vi "MwE with Feeder-.vi"() -> ()   [LabVIEW 2016]
doc: "This example shows how to move a motor connected to an encoder and a wheel, and then read information about the system from an encoder.\n\nThis is an example of how to use feedback (from the encoder) to create an open loop system. If some control method was used, for example using PID, a closed loop system could be created.\n\nThis example expects a USB cable connected from your development PC to the Type B USB Jack (next to the power input) on the roboRIO.\n\nThis example requires the Driver Station to be running with Teleoperated Enabled."
uses:
  <vilib>/Rock Robotics/SystemInterfaces/DIO/FPGA_DIOChannel.ctl
  <vilib>/Rock Robotics/WPI/Encoder/WPI_EncoderType.ctl
  <vilib>/Rock Robotics/SystemInterfaces/DIO/FPGA_DIOPWMChannel.ctl
  <vilib>/Rock Robotics/WPI/MotorControl/WPI_MotorControlOpen SPARK.vi
  <vilib>/Rock Robotics/WPI/Counter/WPI_CounterDigitalInputToDigitalSource.vi
  <vilib>/gmath/NI_Gmath.lvlib
panel:
  in  "Feeder Enabled":bool=TRUE
  out "RPM F":cluster{dbl, dbl}[](graph)
  in  "Motor PWM Channel F":T1=enum."PWM 8"
  in  "Number Samples to Average F":u8=1 min=1 max=128
  in  "Invert Direction F":bool=TRUE
  in  "Decoding Type F":T2=enum."2x"
  in  "DistancePerCount (deg) F":dbl=0.351563
  in  "Encoder B Channel F":T3=enum."DIO 3"
  in  "Encoder A Channel F":T3=enum."DIO 2"
  in  "Minimum Rate F":dbl=20.0
  in  "Update RPM F":bool
  in  "Target RPM F":dbl=770.0
  out "DS Original F":dbl=0.6428571428571428
  in  "Lower Limit F":dbl=-50.0 format="%#_13g"
  in  "Upper Limit F":dbl=50.0 format="%#_13g"
  in  "Pos Drive Signal F":dbl=0.4
  in  "Neg Drive Signal F":dbl=0.05
  out "Error F":dbl(graph)=-19.827905182603445
  out "Error F":dbl=-19.827905182603445
  out "RPM F":dbl=3319.8279051826034
  out "RPM F":dbl(graph)=3319.8279051826034
  out "Encoder Alarm Status F":string="Encoder Moving"
  out "Encoder Direction F":string="Forward"
  in  "Encoder Before Gearbox":bool
  in  "Update RPM L":bool
  in  "Lower Limit L":dbl=-50.0 format="%#_13g"
  in  "Upper Limit L":dbl=50.0 format="%#_13g"
  out "Error L":dbl(graph)=-19.827905182603445
  out "Error L":dbl=-19.827905182603445
  out "DS Original L":dbl=0.6428571428571428
  in  "Neg Drive Signal":dbl=0.6
  in  "Pos Drive Signal":dbl=1.0
  in  "Target RPM":dbl=3300.0
  in  "MS to Wait":u32=10
  out "Loop Time (s)":dbl=0.010378 format="%_6f"
  out "RPM L":dbl=3319.8279051826034
  out "RPM":cluster{dbl[], dbl[]}[](graph)
  out "RPM L":dbl(graph)=3319.8279051826034
  in  "Motor PWM Channel":T1=enum."PWM 9"
  in  "Number Samples to Average":u8=1 min=1 max=128
  in  "Invert Direction L":bool=TRUE
  in  "Decoding Type":T2=enum."2x"
  in  "DistancePerCount (deg)":dbl=0.351563
  in  "Encoder B Channel":T3=enum."DIO 1"
  in  "Encoder A Channel":T3
  in  "Minimum Rate":dbl=20.0
  in  "Stop":bool
  out "Encoder Alarm Status L":string="Encoder Moving"
  out "Encoder Direction L":string="Forward"
  # "These can be set while running."
  # "Output information."
  # "Set these inputs before running."
  # "This example requires the Driver Station to be running with Teleoperated Enabled."
  # "Need to tune target RPM and drive signals"
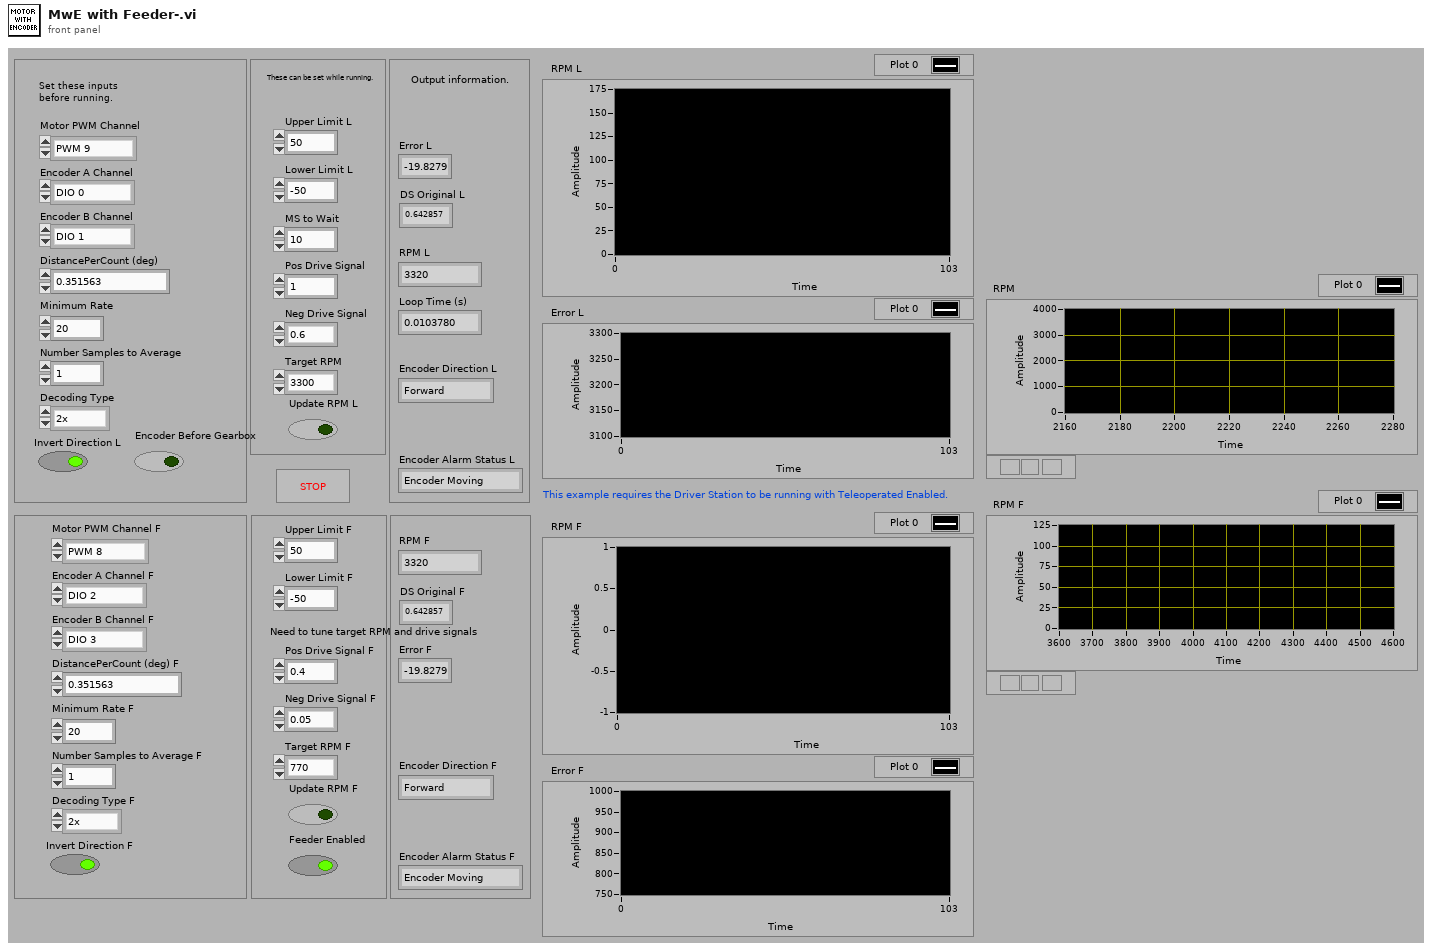
[diagram p1: front panel]
types:
  T1 = typedef "FPGA_DIOPWMChannel.ctl" = enum8{"PWM 0", "PWM 1", "PWM 2", "PWM 3", "PWM 4", "PWM 5", "PWM 6", "PWM 7", "PWM 8", "PWM 9", "PWM MXP 0", "PWM MXP 1", "PWM MXP 2", "PWM MXP 3", "PWM MXP 4", "PWM MXP 5", "PWM MXP 6", "PWM MXP 7", "PWM MXP 8", "PWM MXP 9", "Invalid"}
  T2 = typedef "WPI_EncoderType.ctl" = enum16{"1x", "2x", "4x"}
  T3 = typedef "FPGA_DIOChannel.ctl" = enum8{"DIO 0", "DIO 1", "DIO 2", "DIO 3", "DIO 4", "DIO 5", "DIO 6", "DIO 7", "DIO 8", "DIO 9", "DIO MXP 0", "DIO MXP 1", "DIO MXP 2", "DIO MXP 3", "DIO MXP 4", "DIO MXP 5", "DIO MXP 6", "DIO MXP 7", "DIO MXP 8", "DIO MXP 9", "DIO MXP 10", "DIO MXP 11", "DIO MXP 12", "DIO MXP 13", "DIO MXP 14", "DIO MXP 15", "SPI Port CS1", "SPI Port CS2", "SPI Port CS3", "SPI Port MISO", "SPI Port MOSI", "Invalid"}
  T4 = typedef "WPI_DigitalInputDevRef.ctl" = cluster{"DevStatus":errorcluster, "DIO Channel":T3}
  T5 = typedef "WPI_MotorControlDeviceRef.ctl" = cluster{"DeviceStatus":errorcluster, "Type":T6, "PWM":cluster{"PWM Channel":T1, "DeadBand":T7}, "CAN":cluster{"Device Number":u8, "SetOutput VI Ref":variant, "GetOutput VI Ref":variant, "Enable VI Ref":variant, "Disable VI Ref":variant, "Data":variant}, "Invert":bool}
  T6 = typedef "WPI_MotorControlType.ctl" = enum16{"PWM", "CAN"}
  T7 = typedef "WPI_PWMDeadband.ctl" = cluster{"Name":string, "maxPositivePwm":i32, "minPositivePwm":i32, "centerPwm":i32, "maxNegativePwm":i32, "minNegativePwm":i32, "angularRange":u16}
  T8 = typedef "FPGA_CounterEncoderSourceConvertionLVSourceType.ctl" = cluster{"DevStatus":errorcluster, "AnalogTriggerMode?":bool, "DigitalMode":cluster{"DIO Channel":T9}, "AnalogTriggerMode":cluster{"AnalogTriggerIndex":T10, "OutputType":T11}}
  T9 = typedef "FPGA_DIODigitalSourceChannel.ctl" = enum8{"DIO 0", "DIO 1", "DIO 2", "DIO 3", "DIO 4", "DIO 5", "DIO 6", "DIO 7", "DIO 8", "DIO 9", "DIO MXP 0", "DIO MXP 1", "DIO MXP 2", "DIO MXP 3", "DIO MXP 4", "DIO MXP 5", "DIO MXP 6", "DIO MXP 7", "DIO MXP 8", "DIO MXP 9", "DIO MXP 10", "DIO MXP 11", "DIO MXP 12", "DIO MXP 13", "DIO MXP 14", "DIO MXP 15", "Disabled"}
  T10 = typedef "FPGA_AnalogTriggerIndex.ctl" = enum8{"Trig 0", "Trig 1", "Trig 2", "Trig 3", "Trig 4", "Trig 5", "Trig 6", "Trig 7", "Invalid"}
  T11 = typedef "FPGA_AnalogTriggerOutType.ctl" = enum16{"InWindow", "TriggerState", "Rising", "Falling"}
  T12 = typedef "WPI_EncoderDevRef.ctl" = cluster{"DevStatus":errorcluster, "EncoderIndex":T13, "CounterIndex":T14, "DistancePerCount":dbl, "Decoding Type":T2}
  T13 = typedef "FPGA_EncoderIdx.ctl" = enum8{"Enc 0", "Enc 1", "Enc 2", "Enc 3", "Enc 4", "Enc 5", "Enc 6", "Enc 7", "Invalid"}
  T14 = typedef "FPGA_CounterCtrSystemIndex.ctl" = enum8{"Ctr 0", "Ctr 1", "Ctr 2", "Ctr 3", "Ctr 4", "Ctr 5", "Ctr 6", "Ctr 7", "Invalid"}
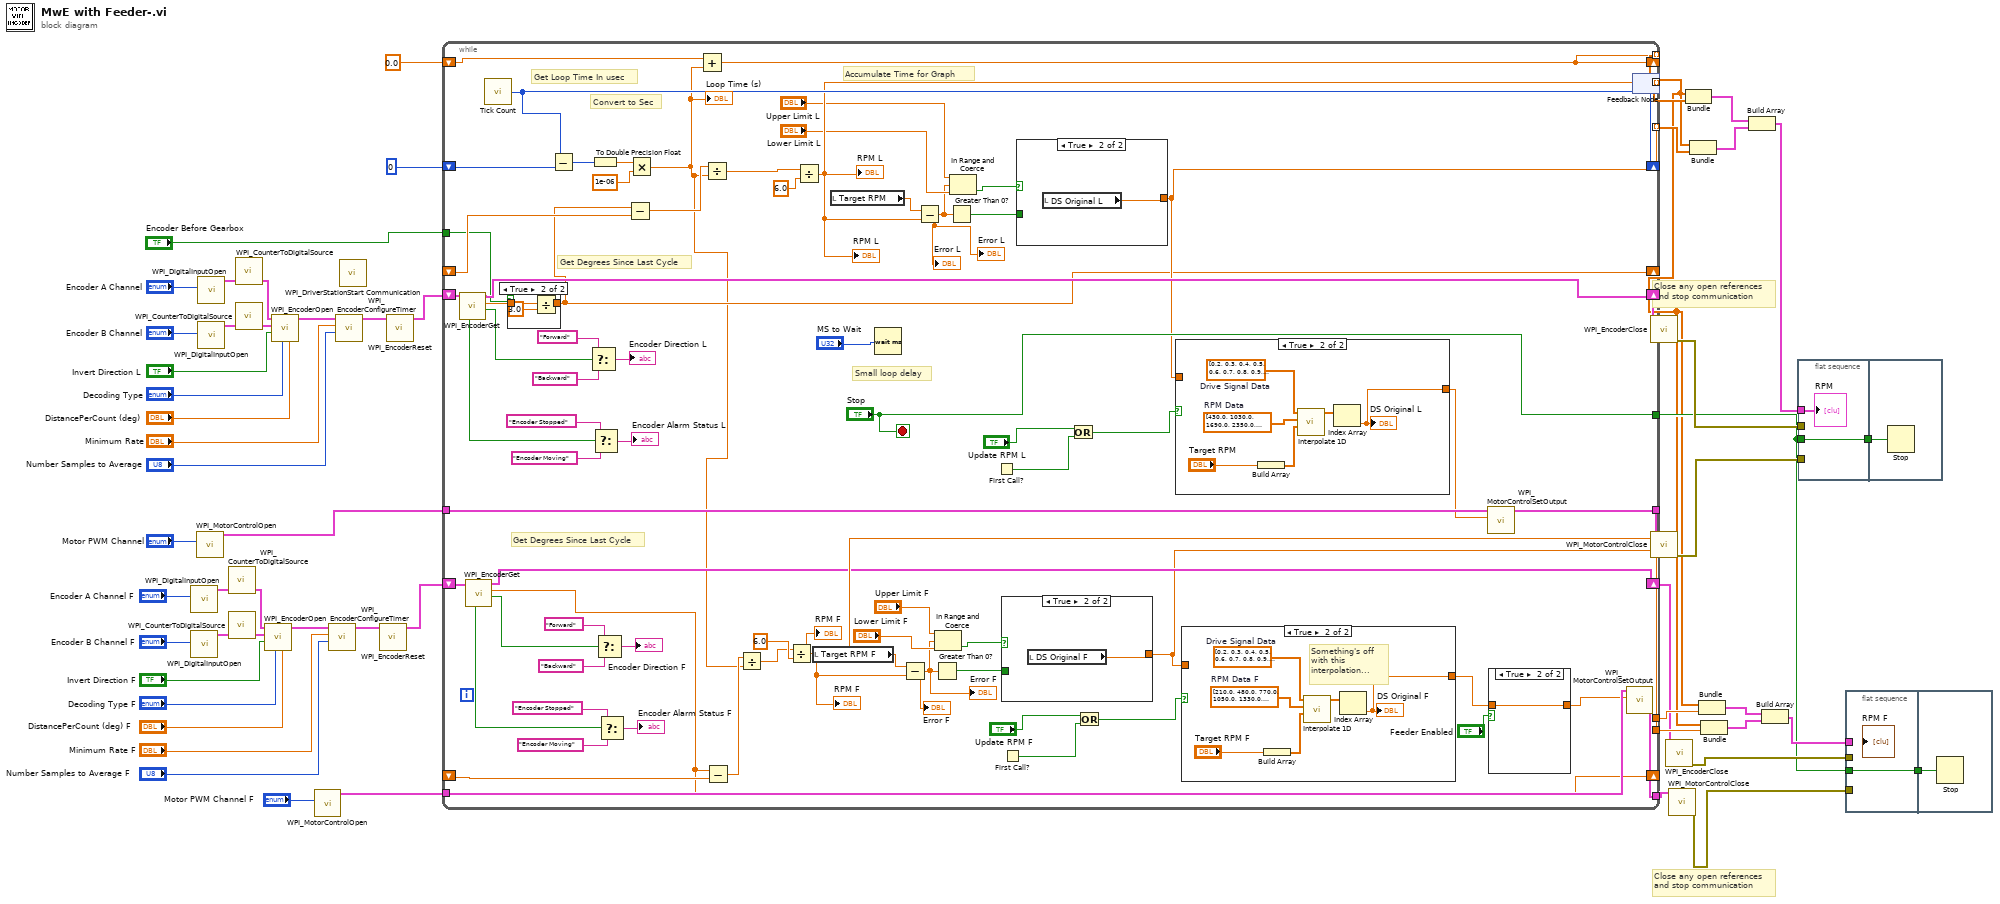
[diagram p0: block diagram]
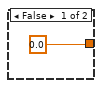
[diagram p2: hidden frame]
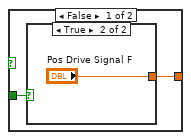
[diagram p4: hidden frame]
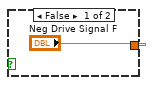
[diagram p5: hidden frame]
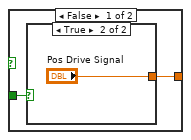
[diagram p8: hidden frame]
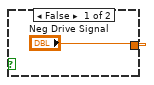
[diagram p9: hidden frame]
diagram:
  # "Close any open references\nand stop communication"
  # "Close any open references\nand stop communication"
  n1 = call <vilib>:"WPI_DigitalInputOpen.vi"("DIO Channel"="Encoder A Channel F") -> ("DigitalInputDevRef"=w27:T4)  [unwired: 1 in, 9 out]
  n2 = call <vilib>:"WPI_DigitalInputOpen.vi"("DIO Channel"="Encoder B Channel F") -> ("DigitalInputDevRef"=w28:T4)  [unwired: 1 in, 9 out]
  n3 = call-poly <vilib>:"WPI_MotorControlOpen.vi"("PWM Channel"="Motor PWM Channel") -> ("MotorControlDeviceRef"=w31:T5)  [unwired: 3 in, 7 out]
  n4 = call <vilib>:"WPI_DigitalInputOpen.vi"("DIO Channel"="Encoder A Channel") -> ("DigitalInputDevRef"=w55:T4)  [unwired: 1 in, 9 out]
  n5 = call <vilib>:"WPI_DigitalInputOpen.vi"("DIO Channel"="Encoder B Channel") -> ("DigitalInputDevRef"=w56:T4)  [unwired: 1 in, 9 out]
  n6 = call-poly <vilib>:"WPI_CounterToDigitalSource.vi"("DigitalInputDevRef"=w27) -> ("Digital Source"=w26:T8)  [unwired: 6 out]
  n7 = call-poly <vilib>:"WPI_CounterToDigitalSource.vi"("DigitalInputDevRef"=w28) -> ("Digital Source"=w29:T8)  [unwired: 6 out]
  n8 = call-poly <vilib>:"WPI_CounterToDigitalSource.vi"("DigitalInputDevRef"=w55) -> ("Digital Source"=w54:T8)  [unwired: 6 out]
  n9 = call-poly <vilib>:"WPI_CounterToDigitalSource.vi"("DigitalInputDevRef"=w56) -> ("Digital Source"=w57:T8)  [unwired: 6 out]
  n10 = call <vilib>:"WPI_EncoderOpen.vi"("DistancePerCount"="DistancePerCount (deg) F", "Decoding Type"="Decoding Type F", "Invert Direction (False)"="Invert Direction F", "BSource"=w29, "ASource"=w26) -> ("EncoderDevRef"=w20:T12)  [unwired: 3 in, 3 out]
  n11 = call <vilib>:"WPI_EncoderOpen.vi"("DistancePerCount"="DistancePerCount (deg)", "Decoding Type"="Decoding Type", "Invert Direction (False)"="Invert Direction L", "BSource"=w57, "ASource"=w54) -> ("EncoderDevRef"=w48:T12)  [unwired: 3 in, 3 out]
  n12 = call-poly <vilib>:"WPI_MotorControlOpen.vi"("PWM Channel"="Motor PWM Channel F") -> ("MotorControlDeviceRef"=w15:T5)  [unwired: 3 in, 7 out]
  n13 = call <vilib>:"WPI_EncoderConfigureTimer.vi"("Number Samples to Average"="Number Samples to Average F", "Minimum Rate"="Minimum Rate F", "EncoderDevRef"=w20) -> ("EncoderDevRef"=w16:T12)  [unwired: 1 in, 7 out]
  n14 = call <vilib>:"WPI_EncoderConfigureTimer.vi"("Number Samples to Average"="Number Samples to Average", "Minimum Rate"="Minimum Rate", "EncoderDevRef"=w48) -> ("EncoderDevRef"=w42:T12)  [unwired: 1 in, 7 out]
  n15 = call <vilib>:"WPI_DriverStationStart Communication.vi"() -> ()  [unwired: 2 in, 10 out]
  n16 = call <vilib>:"WPI_EncoderReset.vi"("EncoderDevRef"=w16) -> ("EncoderDevRef"=w14:T12)  [unwired: 1 in, 9 out]
  n17 = call <vilib>:"WPI_EncoderReset.vi"("EncoderDevRef"=w42) -> ("EncoderDevRef"=w41:T12)  [unwired: 1 in, 9 out]
  n18 = while {
    shift-right: [w116] -> w58
    shift-left: w41 -> [w119]
    tunnel: ["Stop"] -> w4
    tunnel: w31 -> [w122]
    tunnel: [w121] -> w45
    tunnel: [w104] -> w43 mode=indexing
    tunnel: [w106] -> w2 mode=indexing
    shift-right: [w115] -> _
    shift-left: u32 0 ("Tick Count(uSec)") -> [w114]
    shift-right: [w92] -> _
    shift-left: _ -> [w113]
    shift-right: [w106] -> _
    shift-left: 0.0 ("Tick Count(uSec)") -> [w107]
    tunnel: [w98] -> w37 mode=indexing
    tunnel: "Encoder Before Gearbox" -> [w91]
    tunnel: [w70] -> w7
    tunnel: w15 -> [w69]
    shift-right: [w67] -> w5
    shift-left: w14 -> [w68]
    shift-right: [w60] -> _
    shift-left: _ -> [w65]
    tunnel: [w66] -> w6
    tunnel: [w64] -> w3
    stop <- "Stop" stop-if-true
    # "Get Degrees Since Last Cycle"
    # "Accumulate Time for Graph"
    # "Get Degrees Since Last Cycle"
    # "Convert to Sec"
    # "Get Loop Time In usec"
    # "Small loop delay"
    n19 = call <vilib>:"WPI_EncoderGet.vi"("EncoderDevRef"=w119) -> ("Direction"=w128:bool, "Distance"=w93:dbl, "EncoderDevRef"=w116:T12, "Stopped"=w127:bool)  [unwired: 1 in, 6 out]
    n20 = call <vilib>:"WPI_EncoderGet.vi"("EncoderDevRef"=w68) -> ("Direction"=w88:bool, "Distance"=w60:dbl, "EncoderDevRef"=w67:T12, "Stopped"=w87:bool)  [unwired: 1 in, 6 out]
    n21 = call "Tick Count"() -> ("Tick Count(uSec)"=w115:u32)
    n22 = case shown="True" w91 {
      tunnel: w93 -> [w145 w148]
      tunnel: [w145 w147] -> w92
      frame False {
      }
      frame True {
        n23 = Divide(x=w148, y=3.0) -> (x/y=w147:dbl)
      }
    }
    n24 = Subtract(x=w115, y=w114) -> (x-y=w112:u32)
    n25 = Select(t="Forward", s=w128, f="Backward") -> (s? t:f=→"Encoder Direction L":string)
    n26 = To Double Precision Float(number=w112) -> (double precision float=w110:dbl)
    n27 = Select(t="Encoder Stopped", s=w127, f="Encoder Moving") -> (s? t:f=→"Encoder Alarm Status L":string)
    n28 = Select(t="Forward", s=w88, f="Backward") -> (s? t:f=→"Encoder Direction F":string)
    n29 = Select(t="Encoder Stopped", s=w87, f="Encoder Moving") -> (s? t:f=→"Encoder Alarm Status F":string)
    n30 = Subtract(x=w92, y=w113) -> (x-y=w109:dbl)
    n31 = Multiply(x=w110, y=1e-06) -> (x*y=w59:dbl)
    "Loop Time (s)" <- w59
    n32 = Add(x=w107, y=w59) -> (x+y=w106:dbl)
    n33 = Divide(x=w109, y=w59) -> (x/y=w108:dbl)
    n34 = Subtract(x=w60, y=w65) -> (x-y=w81:dbl)
    n35 = Divide(x=w81, y=w59) -> (x/y=w80:dbl)
    n36 = Divide(x=w80, y=6.0) -> (x/y=w70:dbl)
    "RPM F" <- w70
    "RPM F" <- w70
    n37 = Divide(x=w108, y=6.0) -> (x/y=w104:dbl)
    "RPM L" <- w104
    "RPM L" <- w104
    n38 = local read "Target RPM F"() -> (w79:dbl)
    n39 = local read "Target RPM"() -> (w105:dbl)
    n40 = Wait (ms)(milliseconds to wait="MS to Wait") -> ()  [unwired: 1 out]
    n41 = Subtract(x=w79, y=w70) -> (x-y=w74:dbl)
    "Error F" <- w74
    "Error F" <- w74
    n42 = Subtract(x=w105, y=w104) -> (x-y=w99:dbl)
    "Error L" <- w99
    "Error L" <- w99
    n43 = Greater Than 0?(x=w74) -> (x > 0?=w78:bool)
    n44 = In Range and Coerce(upper limit="Upper Limit F", x=w74, lower limit="Lower Limit F") -> (In Range?=w75:bool)  [unwired: 1 out]
    n45 = Greater Than 0?(x=w99) -> (x > 0?=w103:bool)
    n46 = In Range and Coerce(upper limit="Upper Limit L", x=w99, lower limit="Lower Limit L") -> (In Range?=w100:bool)  [unwired: 1 out]
    n47 = First Call?() -> (First Call?: T/F=w94:bool)
    n48 = First Call?() -> (First Call?: T/F=w71:bool)
    n49 = case shown="True" w75 {
      tunnel: w78 -> [w141 _]
      tunnel: [w140 w144] -> w66
      frame False {
        n50 = case shown="True" w141 {
          tunnel: ["Neg Drive Signal F" "Pos Drive Signal F"] -> w140
          frame False {
          }
          frame True {
          }
        }
      }
      frame True {
        n51 = local read "DS Original F"() -> (w144:dbl)
      }
    }
    n52 = case shown="True" w100 {
      tunnel: w103 -> [w157 _]
      tunnel: [w156 w160] -> w98
      frame False {
        n53 = case shown="True" w157 {
          tunnel: ["Neg Drive Signal" "Pos Drive Signal"] -> w156
          frame False {
          }
          frame True {
          }
        }
      }
      frame True {
        n54 = local read "DS Original L"() -> (w160:dbl)
      }
    }
    n55 = Or(x="Update RPM L", y=w94) -> (x .or. y?=w95:bool)
    n56 = Or(x="Update RPM F", y=w71) -> (x .or. y?=w72:bool)
    n57 = case shown="True" w95 {
      tunnel: [w149 w150] -> w97
      tunnel: w98 -> [w149 _]
      frame False {
      }
      frame True {
        w155 = dbl[] [430.0, 1030.0, 1690.0, 2350.0, 3000.0, 3700.0, 4400.0, 5000.0, 5550.0]  # RPM Data
        w154 = dbl[] [0.2, 0.3, 0.4, 0.5, 0.6, 0.7, 0.8, 0.9, 1.0]  # Drive Signal Data
        n58 = Build Array("Target RPM") -> (w152:dbl[])
        n59 = call <vilib>:"Interpolate 1D.vi"("xi"=w152, "X"=w155, "Y"=w154) -> ("yi"=w151:dbl[])  [unwired: 6 in, 2 out]
        n60 = Index Array(array=w151) -> (element=w150:dbl)  [unwired: 1 in]
        "DS Original L" <- w150
      }
    }
    n61 = case shown="True" w72 {
      tunnel: [w133 w134] -> w63
      tunnel: w66 -> [w133 _]
      frame False {
      }
      frame True {
        w139 = dbl[] [210.0, 480.0, 770.0, 1050.0, 1330.0, 1650.0, 1870.0, 2140.0, 2400.0]  # RPM Data F
        w138 = dbl[] [0.2, 0.3, 0.4, 0.5, 0.6, 0.7, 0.8, 0.9, 1.0]  # Drive Signal Data
        # "Something's off \nwith this\ninterpolation..."
        n62 = Build Array("Target RPM F") -> (w136:dbl[])
        n63 = call <vilib>:"Interpolate 1D.vi"("xi"=w136, "X"=w139, "Y"=w138) -> ("yi"=w135:dbl[])  [unwired: 6 in, 2 out]
        n64 = Index Array(array=w135) -> (element=w134:dbl)  [unwired: 1 in]
        "DS Original F" <- w134
      }
    }
    n65 = call <vilib>:"WPI_MotorControlSetOutput.vi"("Output"=w97, "MotorControlDevRef"=w122) -> ("MotorControlDevRef"=w121:T5)  [unwired: 2 in, 7 out]
    n66 = case shown="True" "Feeder Enabled" {
      tunnel: [0.0 w132] -> w62
      tunnel: w63 -> [_ w132]
      frame False {
      }
      frame True {
      }
    }
    n67 = call <vilib>:"WPI_MotorControlSetOutput.vi"("Output"=w62, "MotorControlDevRef"=w69) -> ("MotorControlDevRef"=w64:T5)  [unwired: 2 in, 7 out]
  }
  n68 = feedback-in #1(w2) -> ()
  n69 = feedback #1() -> (w1:dbl[])  [unwired: 1 in]
  n70 = call <vilib>:"WPI_EncoderClose.vi"("EncoderDevRef"=w58) -> ("error out"=w33:errorcluster)  [unwired: 2 in, 8 out]
  n71 = call <vilib>:"WPI_MotorControlClose.vi"("MotorControlDevRef"=w45) -> ("error out"=w32:errorcluster)  [unwired: 1 in, 9 out]
  n72 = call <vilib>:"WPI_EncoderClose.vi"("EncoderDevRef"=w5) -> ("error out"=w9:errorcluster)  [unwired: 2 in, 8 out]
  n73 = call <vilib>:"WPI_MotorControlClose.vi"("MotorControlDevRef"=w3) -> ("error out"=w8:errorcluster)  [unwired: 1 in, 9 out]
  n74 = Bundle(w1, w43) -> (w36:cluster{dbl[], dbl[]})  [unwired: 1 in]
  n75 = Bundle(w1, w37) -> (w35:cluster{dbl[], dbl[]})  [unwired: 1 in]
  n76 = Bundle(w1, w7) -> (w12:cluster{dbl[], dbl})  [unwired: 1 in]
  n77 = Bundle(w1, "DS Original F"=w6) -> (w11:cluster{dbl[], "DS Original F":dbl})  [unwired: 1 in]
  n78 = Build Array(w36, w35) -> (w34:cluster{dbl[], dbl[]}[])
  n79 = Build Array(w12, w11) -> (w10:cluster{dbl[], "DS Original F":dbl}[])
  n80 = flat-sequence {
    tunnel: w4 -> [w162]
    tunnel: [w162] -> w40
    tunnel: w34 -> [w161]
    tunnel: w33 -> [_]
    tunnel: w32 -> [_]
    tunnel: w40 -> [w163]
    frame #0 {
      "RPM" <- w161
    }
    frame #1 {
      n81 = Stop(stop? (T)=w163) -> ()
    }
  }
  n82 = flat-sequence {
    tunnel: w4 -> [w164]
    tunnel: [w164] -> w13
    tunnel: w10 -> [_]
    tunnel: w9 -> [_]
    tunnel: w8 -> [_]
    tunnel: w13 -> [w165]
    frame #0 {
    }
    frame #1 {
      n83 = Stop(stop? (T)=w165) -> ()
    }
  }
